vi "DELETETest Sweep.vi"(8 "error in (no error)":errorcluster, 11 "Lockin.DAQ in":refnum<class "Instrument.DAQ.lvclass">) -> (0 "error out":errorcluster, 3 "Lockin.DAQ out":refnum<class "Instrument.DAQ.lvclass">)   [LabVIEW 2019]
uses:
  Instrument.DAQ.lvclass
  Typedefs/AO.Channel--Cluster--Array.ctl
  Typedefs/AO.Channel--Cluster.ctl
  Typedefs/AO.Channel.Function--Enum.ctl
  Waveguide Model/Waveguide Model--Cluster.ctl
  Typedefs/DAQ.Sampling.Sampling--Cluster.ctl
  Typedefs/REF.Channel--Cluster--Array.ctl
  Typedefs/REF.Channel--Cluster.ctl
  Typedefs/AI.Channel--Cluster--Array.ctl
  Typedefs/AI.Channel--Cluster.ctl
  Instrument.DAQ.lvclass/Instrument.DAQ.ctl
  <vilib>/Analysis/baseanly.llb/Mean (DBL).vi
  <vilib>/Analysis/NI_AALBase.lvlib
  C:/Program Files/National Instruments/LabVIEW 2019/vi.lib/JKI/JKI SMO/SMO/SMO.lvclass
panel:
  in  "Configuration.AI Channels":T1 {"References" items=["", "1", "2", "3"]; "Channel" min=1}
  in  "Configuration.Channels: REF":T3 {"Roll-Off" min=1; "TC" min=0.0001 format="%#_3p"; "Phase" format="%.3g"; "Frequency" min=0.0001 max=10000.0 format="%.3g"; "Channel" min=1}
  in  "sampling":T5={"Fs"=204789.0, "#s"=15753} {"Fs" format="%#_13g"}
  in  "Enum":enum16{"X", "Y", "R", "Theta", "Mean"}(ring)
  in  "stop":bool
  in  "Simulate Waveguide":bool
  out "Average time (ms)":dbl=0.328125
  in  "Waveguide Cluster":T6
  out "Waveform Chart 2":u32(graph)
  out "Waveform Chart":dbl[][](graph)=[[-0.22911635604378638]]
  in  "AO Chanels":T7=[{"Enable?"=FALSE, "Channel"=0, "Amplitude"=0.0, "Offset"=0.0, "Frequency"=0.1, "Phase"=0.0, "Function"=enum."Sine", "Sweeping?"=FALSE}] {"Phase" format="%.3g"; "Frequency" min=0.0001 max=10000.0 format="%.3g"; "Offset" format="%.3p"; "Amplitude" min=0.0 max=10.0 format="%.3p"}
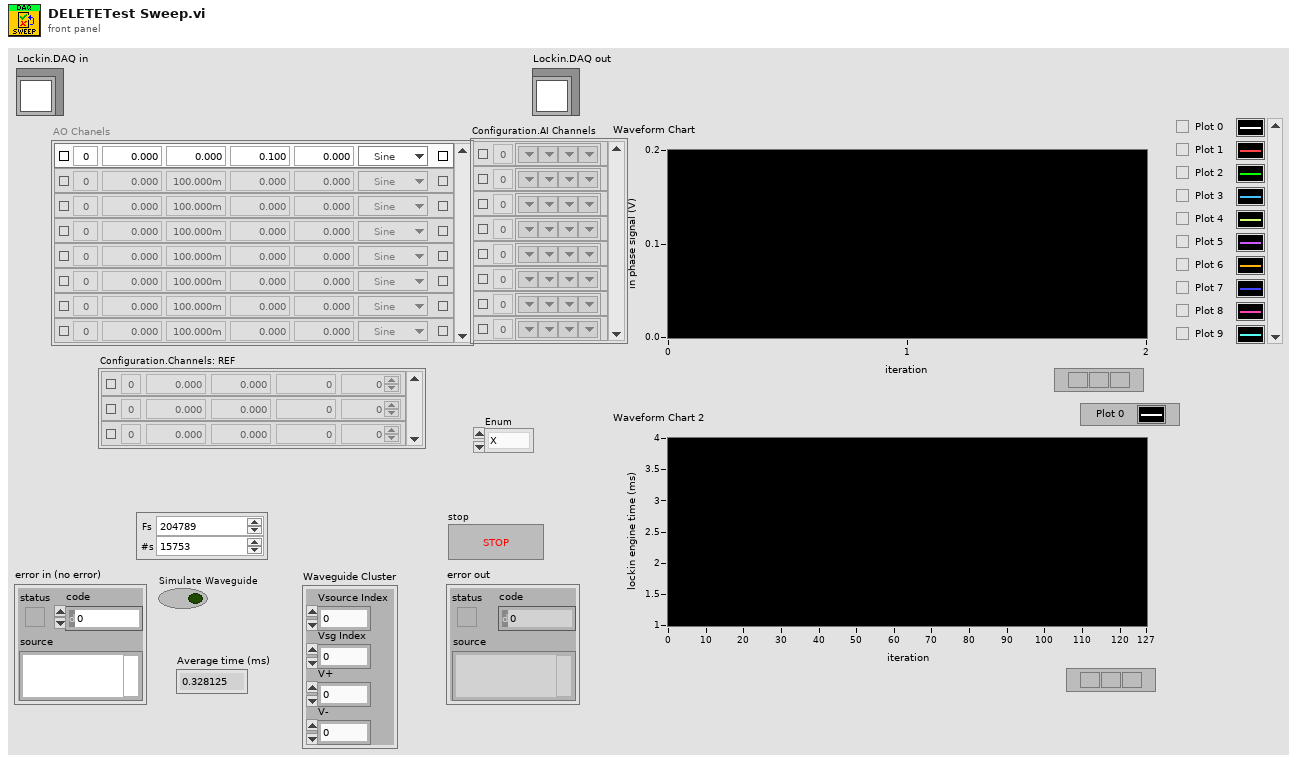
[diagram p1: front panel]
types:
  T1 = typedef "Instrument.Lockin.lvlib/Instrument.DAQ.lvclass/AI.Channel--Cluster--Array.ctl" = T2[]
  T2 = typedef "Instrument.Lockin.lvlib/Instrument.DAQ.lvclass/AI.Channel--Cluster.ctl" = cluster{"Enable?":bool, "Channel":i32, "References":i32[]}
  T3 = typedef "Instrument.Lockin.lvlib/Instrument.DAQ.lvclass/REF.Channel--Cluster--Array.ctl" = T4[]
  T4 = typedef "Instrument.Lockin.lvlib/Instrument.DAQ.lvclass/REF.Channel--Cluster.ctl" = cluster{"Enable?":bool, "Channel":i32, "Frequency":dbl, "Phase":dbl, "TC":dbl, "Roll-Off":i32}
  T5 = typedef "Instrument.Lockin.lvlib/Instrument.DAQ.lvclass/DAQ.Sampling.Sampling--Cluster.ctl" = cluster{"Fs":dbl, "#s":i32}
  T6 = typedef "Instrument.Lockin.lvlib/Instrument.DAQ.lvclass/Waveguide Model--Cluster.ctl" = cluster{"Vsource Index":i32, "Vsg Index":i32, "V+":i32, "V-":i32}
  T7 = typedef "Instrument.Lockin.lvlib/Instrument.DAQ.lvclass/AO.Channel--Cluster--Array.ctl" = T8[]
  T8 = typedef "Instrument.Lockin.lvlib/Instrument.DAQ.lvclass/AO.Channel--Cluster.ctl" = cluster{"Enable?":bool, "Channel":i32, "Amplitude":dbl, "Offset":dbl, "Frequency":dbl, "Phase":dbl, "Function":T9, "Sweeping?":bool}
  T9 = typedef "Instrument.Lockin.lvlib/Instrument.DAQ.lvclass/AO.Channel.Function--Enum.ctl" = enum16{"Sine", "Triangle", "Square"}
  T10 = typedef "Instrument.Lockin.lvlib/Instrument.DAQ.lvclass/Results--Cluster.ctl" = cluster{"Time Stamp":timestamp, "Results (Dictionary)":cluster{"key":string, "value":dbl}[]}
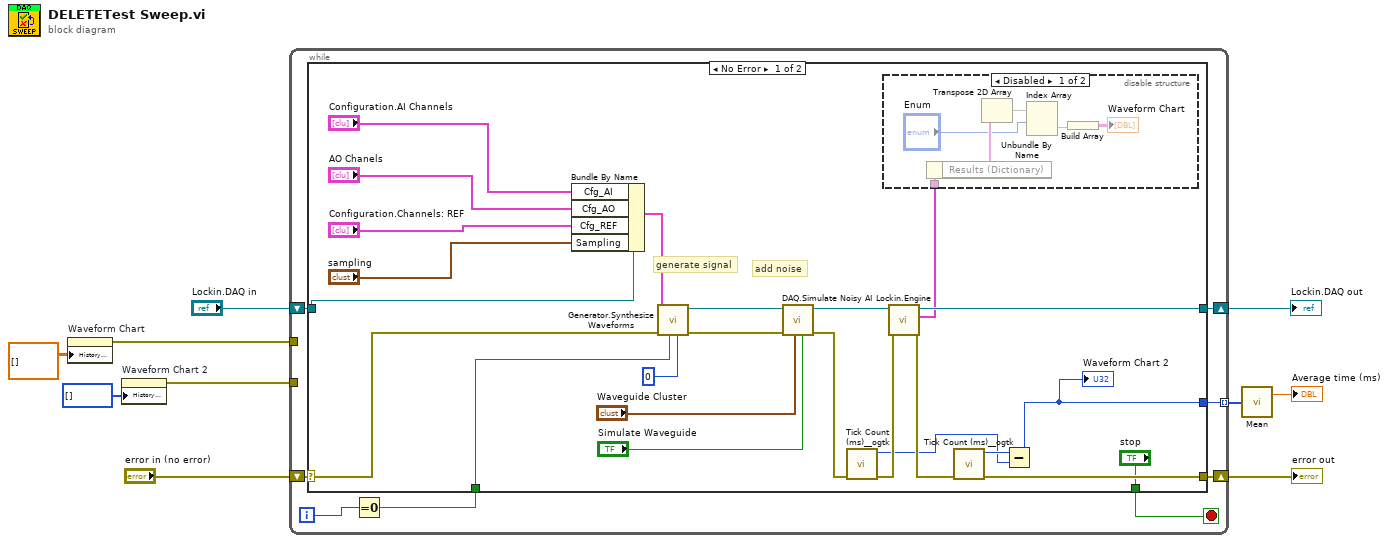
[diagram p0: block diagram]
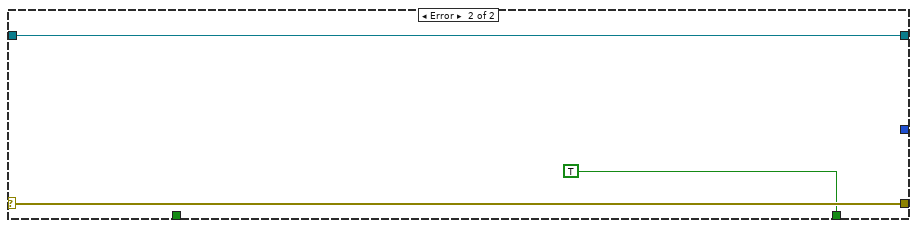
[diagram p3: hidden frame]
diagram:
  n1 = property on="Waveform Chart" class="WFChart (strict)"("History Data"=dbl[][] []) -> (error out=w2:errorcluster)  [unwired: 2 in, 1 out]
  n2 = property on="Waveform Chart 2" class="WFChart (strict)"("History Data"=u32[] []) -> (error out=w3:errorcluster)  [unwired: 2 in, 1 out]
  n3 = while {
    shift-right: [w17] -> w9
    shift-left: "error in (no error)" -> [w18]
    shift-right: [w15] -> w7
    shift-left: "Lockin.DAQ in" -> [w16]
    tunnel: [w14] -> w4 mode=indexing
    tunnel: w3 -> [_]
    tunnel: w2 -> [_]
    i -> [w12]
    stop <- w11 stop-if-true
    n4 = Equal To 0?(x=w12) -> (x = 0?=w13:bool)
    n5 = case shown="No Error" w18 {
      selector: w18 -> [w40 w51]
      tunnel: [w34 w51] -> w17
      tunnel: [w38 w50] -> w15
      tunnel: w16 -> [w20 w50]
      tunnel: [w32 _] -> w14
      tunnel: w13 -> [w29 _]
      tunnel: ["stop" TRUE ("stop")] -> w11
      frame No Error {
        # "generate signal"
        # "add noise"
        n6 = Bundle By Name(cluster=w20, "Cfg_AI"="Configuration.AI Channels", "Cfg_AO"="AO Chanels", "Cfg_REF"="Configuration.Channels: REF", "Sampling"="sampling") -> (w21:cluster{})
        n7 = call "Generator.Synthesize Waveforms.vi"("sweep state"=0 ("sweep index"), "Reset Phase?"=w29, "error in (no error)"=w40, "Instrument.DAQ"=w21) -> ("error out"=w41:errorcluster, "Instrument.DAQ"=w42:refnum<class "Instrument.DAQ.lvclass">)  [unwired: 6 in]
        n8 = call "DAQ.Simulate Noisy AI.vi"("Simulate Waveguide [T]"="Simulate Waveguide", "Waveguide Cluster"="Waveguide Cluster", "error in (no error)"=w41, "Instrument.DAQ in"=w42) -> ("error out"=w36:errorcluster, "Instrument.DAQ out"=w39:refnum<class "Instrument.DAQ.lvclass">)  [unwired: 6 in]
        n9 = call <userlib>:"Tick Count (ms)__ogtk.vi"("error in (no error)"=w36) -> ("error out"=w35:errorcluster, "millisecond timer value"=w26:u32)  [unwired: 9 in]
        n10 = call "Lockin.Engine.vi"("error in (no error)"=w35, "Instrument.DAQ"=w39) -> ("error out"=w31:errorcluster, "<Results> (X,Y,R,Theta,Mean)"=w37:T10, "Instrument.DAQ out"=w38:refnum<class "Instrument.DAQ.lvclass">)  [unwired: 7 in]
        n11 = disable-structure shown="Disabled" {
          disable-tunnel: w37 -> [w47 _]
          frame Disabled {
            n12 = Unbundle By Name(w47) -> ("Results (Dictionary)"=w44:cluster{"key":string, "value":dbl}[])
            n13 = Transpose 2D Array(2D array=w44) -> (transposed array=w48:cluster{"key":string, "value":dbl}[][])
            n14 = Index Array(array=w48, index (row)="Enum") -> (element=w46:cluster{"key":string, "value":dbl}[])  [unwired: 1 in]
            n15 = Build Array(w46) -> (→"Waveform Chart":cluster{"key":string, "value":dbl}[][])
          }
          frame Enabled {
          }
        }
        n16 = call <userlib>:"Tick Count (ms)__ogtk.vi"("error in (no error)"=w31) -> ("error out"=w34:errorcluster, "millisecond timer value"=w33:u32)  [unwired: 9 in]
        n17 = Subtract(x=w33, y=w26) -> (x-y=w32:u32)
        "Waveform Chart 2" <- w32
      }
      frame Error {
      }
    }
  }
  "error out" <- w9
  "Lockin.DAQ out" <- w7
  n18 = call-poly <vilib>:"Mean.vi"("X"=w4) -> ("mean"=→"Average time (ms)":dbl)  [unwired: 1 out]
